vi "Main.vi"() -> ()   [LabVIEW 2014]
doc: "This sample project is built upon the standard state machine template and shows how you could create an application that acquires, analyzes, and presents data. It includes functionality for presenting configuration dialogs, preserving settings between executions, loading and saving data, as well as exporting graph images and text files.\n\nIt is most appropriate for data that is acquired instantly as it does not allow for screen updates mid acquisition nor does it allow for continuous streaming to disk."
uses:
  romtests/testproj/controls/DAQSettings.ctl
  romtests/testproj/controls/TriggerMode.ctl
  romtests/testproj/controls/AspicSettings.ctl
  romtests/testproj/controls/AspicMode.ctl
  romtests/testproj/controls/Timeslice.ctl
  romtests/testproj/controls/SystemSet.ctl
  romtests/testproj/controls/Data.ctl
  romtests/testproj/controls/UI References.ctl
  romtests/testproj/controls/Graph Data.ctl
  <vilib>/Utility/miscctls.llb/LVAnnotationListTypeDef.ctl
  <vilib>/Utility/miscctls.llb/LVCursorListTypeDef.ctl
  romtests/testproj/controls/User Specified Data.ctl
  romtests/testproj/controls/HW Configuration.ctl
  romtests/testproj/controls/Simulated Signal Type.ctl
  romtests/testproj/controls/Analysis Configuration.ctl
  romtests/testproj/controls/New Data Behavior.ctl
  romtests/testproj/controls/Network.ctl
  romtests/testproj/controls/CommSelect.ctl
  romtests/testproj/controls/State.ctl
panel:
  out "size(s)":i32[](array[numeric])
  in  "Channel":T1(ring)
  in  "Show":bool
  out "System Set":T2
  in  "SystemSet":bool
  in  "DAQSettings":bool
  in  "Timeslice":bool
  in  "Path settings":bool
  in  "Network Settings":bool
  in  "ASPIC Settings":bool
  in  "Snapshot":bool
  in  "Analyze":bool
  in  "Clear":bool
  in  "Exit":bool
  in  "Acquire":bool
  in  "Export":bool
  in  "Save Data":bool
  in  "Load Data":bool
  in  "Numeric":dbl
  out "timeslice":T3
  out "Aspic Seeting":T4 {"RC" format="%b"; "Gain" format="%b"}
  out "DAQ Settings":T6
  out "Graph":waveform(dbl)[](graph)
  out "Status Bar":string
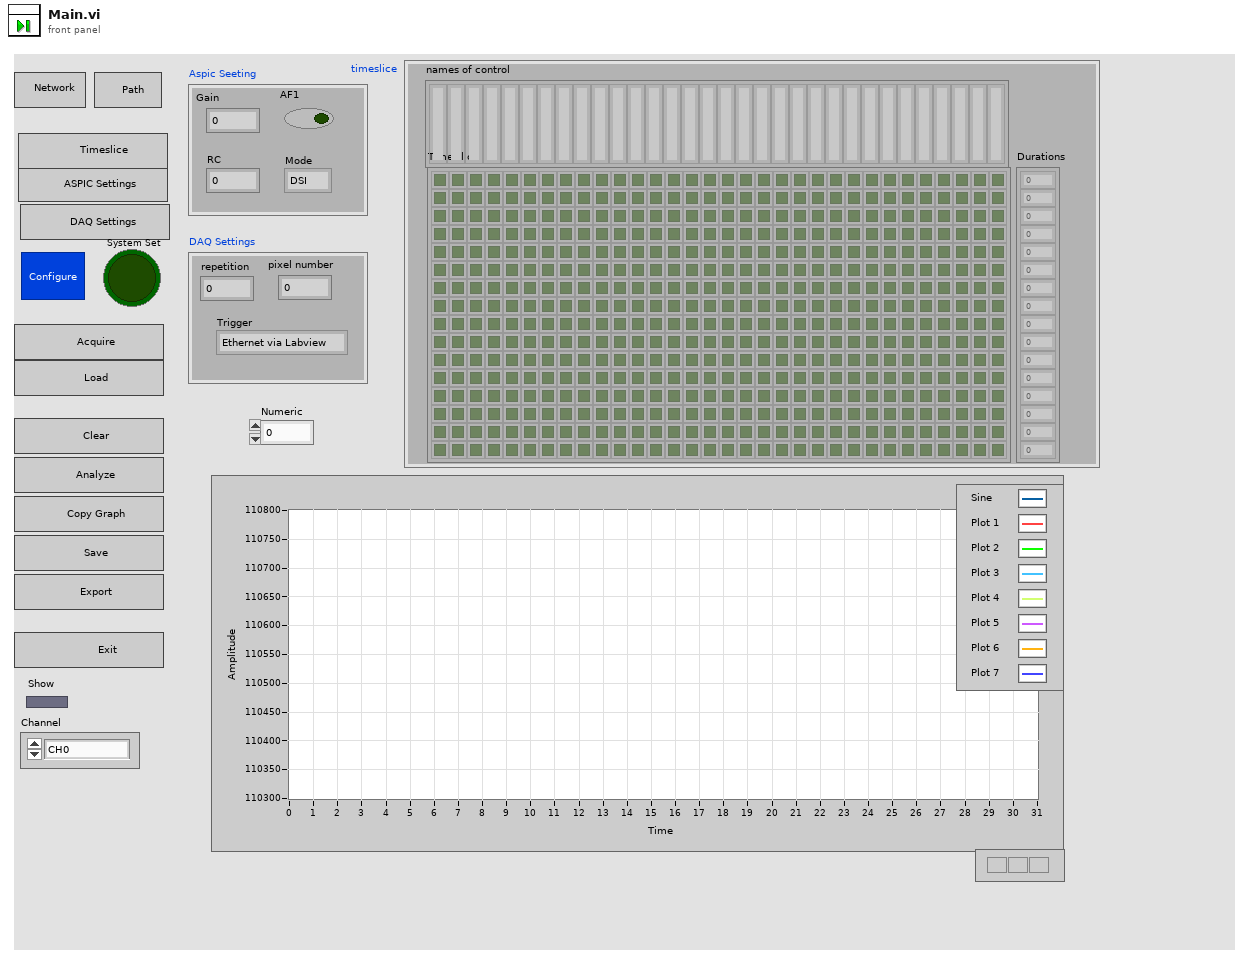
[diagram p1: front panel]
types:
  T1 = enum16{"CH0", "CH1", "CH2", "CH3", "CH4", "CH5", "CH6", "CH7", "All"}
  T2 = typedef "SystemSet.ctl" = bool
  T3 = typedef "Timeslice.ctl" = cluster{"Time slice":bool[][], "Durations":dbl[], "names of control":string[]}
  T4 = typedef "AspicSettings.ctl" = cluster{"Gain":u8, "RC":u8, "aspic1Data":u32[], "aspic2Data":u32[], "AF1":bool, "Mode":T5}
  T5 = typedef "AspicMode.ctl" = enum16{"DSI", "TM"}
  T6 = typedef "DAQSettings.ctl" = cluster{"pixel number":u32, "repetition":u32, "Trigger":T7}
  T7 = typedef "TriggerMode.ctl" = enum16{"Ethernet via Labview", "SMA (1.8V)"}
  T8 = typedef "State.ctl" = enum16{"Initialize", "Wait for Event", "Update UI", "Network", "Configure", "DAQSettings", "Timeslice", "Set Sytem", "Acquire", "Load Data", "Save Data", "Clear Data", "Export Data", "Analyze", "Copy Graph", "Exit"}
  T9 = typedef "Data.ctl" = cluster{"UI References":T10, "Graph Data":T11, "User Specified":T14, "Aspic Seeting":T4, "Network":T19, "timeslice":T3, "Acquisition Settings":T6, "CommSelect":T20, "System Set":T2}
  T10 = typedef "UI References.ctl" = cluster{"Exit Ref":refnum<vi>, "Save Ref":refnum<vi>, "Open Ref":refnum<vi>, "Export Ref":refnum<vi>, "Acquire Ref":refnum<vi>, "Configure Ref":refnum<vi>, "Graph Ref":refnum<vi>, "Clear Ref":refnum<vi>, "Analyze Ref":refnum<vi>, "Status Ref":refnum<vi>, "Snapshot Ref":refnum<vi>, "Network Ref":refnum<vi>, "Timeslice Ref":refnum<vi>, "DAQSetting Ref":refnum<vi>, "SystemSet":refnum<vi>}
  T11 = typedef "Graph Data.ctl" = cluster{"Data":waveform(dbl)[], "Annotation List":T12, "Cursor List":T13, "Analysis Data":waveform(dbl)[]}
  T12 = typedef "LVAnnotationListTypeDef.ctl" = cluster{"Name":string, "Color":u32, "Style":u8, "Point Style":u8, "Name Visible":bool, "Allow Drag":bool, "Annotation Mode":u32, "Plot":i32, "Index":i32, "Position":cluster{"X":dbl, "Y":dbl}, "X Scale":u32, "Y Scale":u32, "Show Arrow":bool, "Lock Name":bool, "Plot Area":i32, "Label Offset":cluster{"X":dbl, "Y":dbl}}[]
  T13 = typedef "LVCursorListTypeDef.ctl" = cluster{"Name":string, "Color":u32, "Style":u8, "Point Style":u8, "Name Visible":bool, "Allow Drag":bool, "Cursor Mode":u32, "Plot":i32, "Index":i32, "Position":cluster{"X":dbl, "Y":dbl}, "X Scale":u32, "Y Scale":u32, "Watch Plots":i32[], "Watch All Plots":bool, "Plot Area":i32, "Label Offset":cluster{"X":dbl, "Y":dbl}}[]
  T14 = typedef "User Specified Data.ctl" = cluster{"Hardware Configuration":T15, "Analysis Configuration":T17, "New Data Behavior":T18}
  T15 = typedef "HW Configuration.ctl" = cluster{"HW Refnum <Replace Me>":string, "Signal Type <Replace Me>":T16}
  T16 = typedef "Simulated Signal Type.ctl" = enum16{"Sine Wave", "Square Wave"}
  T17 = typedef "Analysis Configuration.ctl" = cluster{"Statistics":bool}
  T18 = typedef "New Data Behavior.ctl" = enum16{"Replace", "Overlay", "Append"}
  T19 = typedef "Network.ctl" = cluster{"invert_send":bool, "Number of datagrams to read":u32, "max bytes/read":i32, "Timeout":i32, "host":string, "Port Receive":u16}
  T20 = typedef "CommSelect.ctl" = enum16{"startTSL", "writeCABAC", "readCABAC", "resetCABAC", "emissionTest", "regRead", "executeASPIC", "resetASPIC", "resetFifo18ASPIC", "resetFifo16ASPIC", "LabviewDamicStart"}
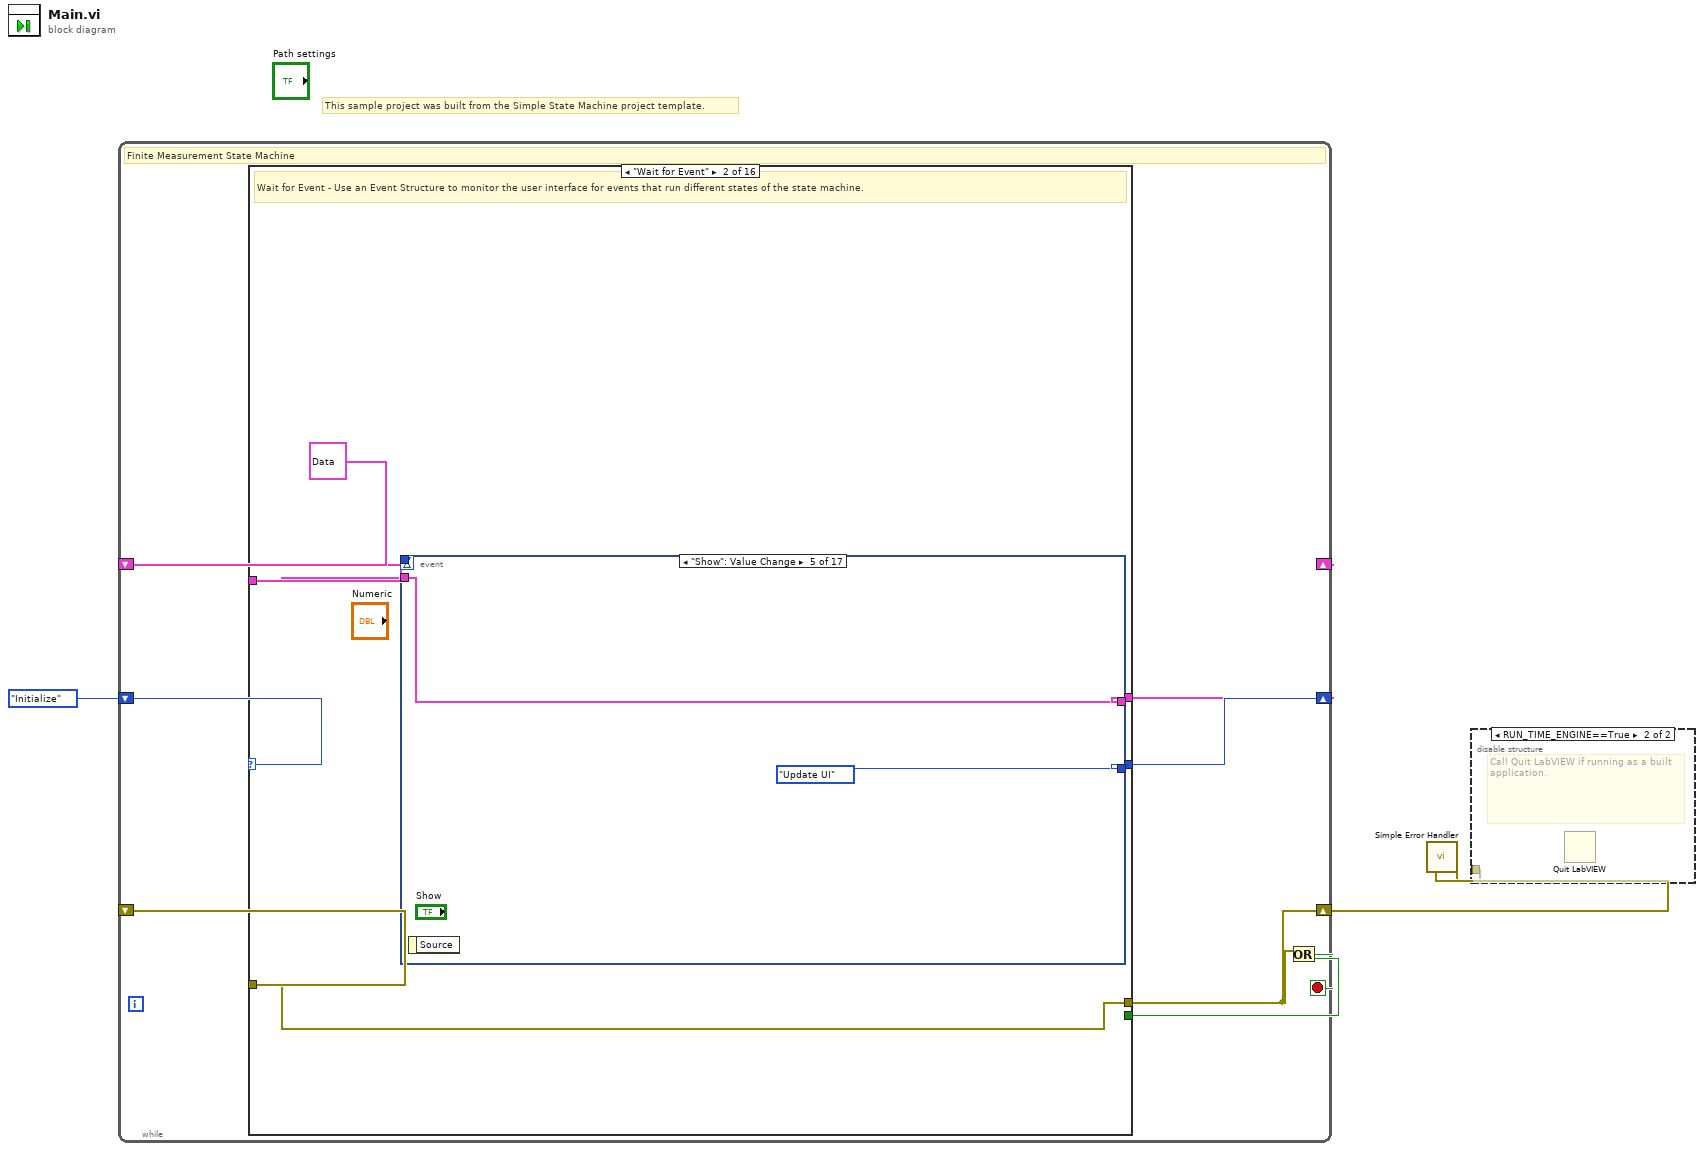
[diagram p0: block diagram]
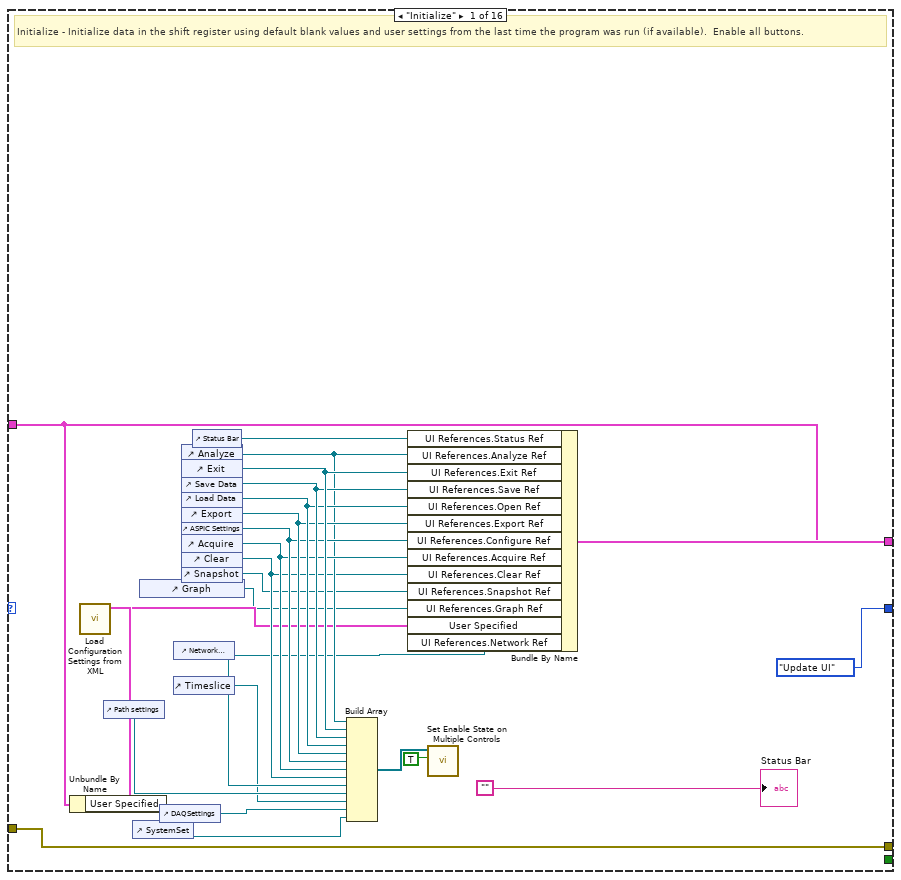
[diagram p3: hidden frame]
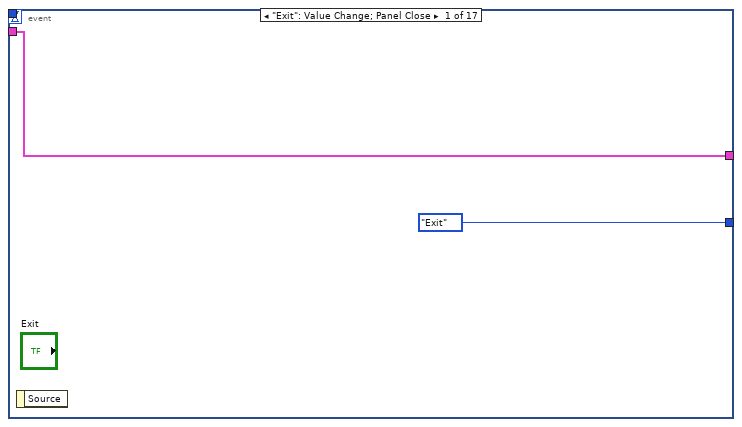
[diagram p4: hidden frame]
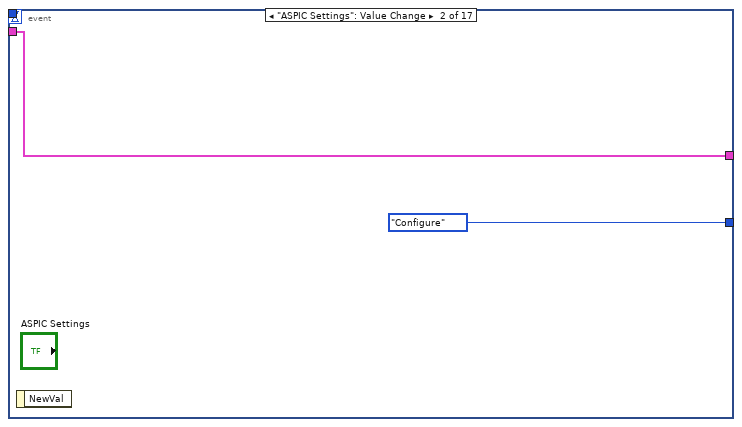
[diagram p5: hidden frame]
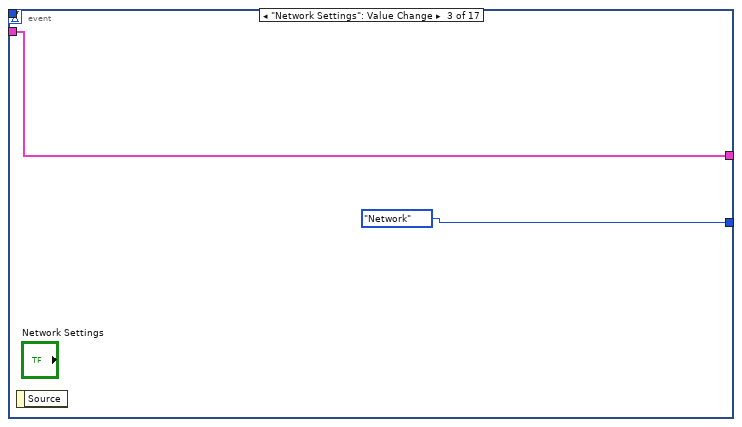
[diagram p6: hidden frame]
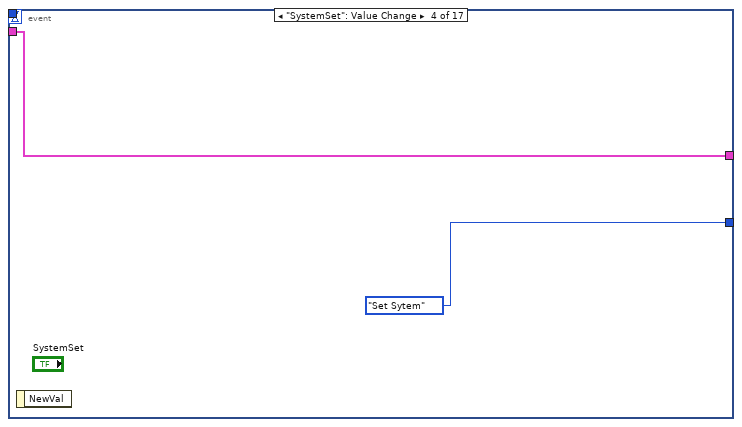
[diagram p7: hidden frame]
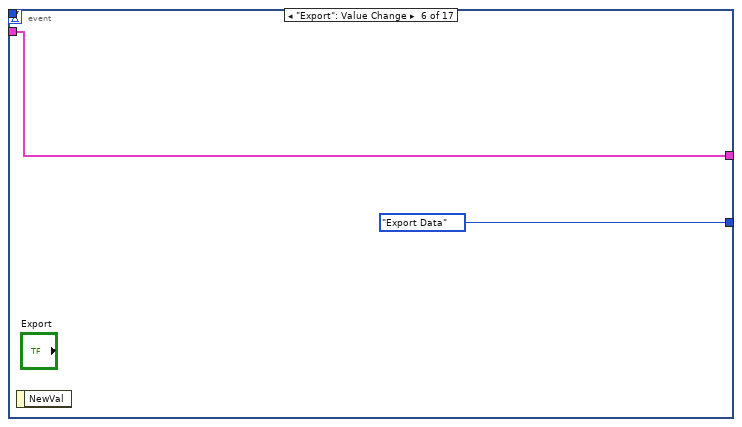
[diagram p8: hidden frame]
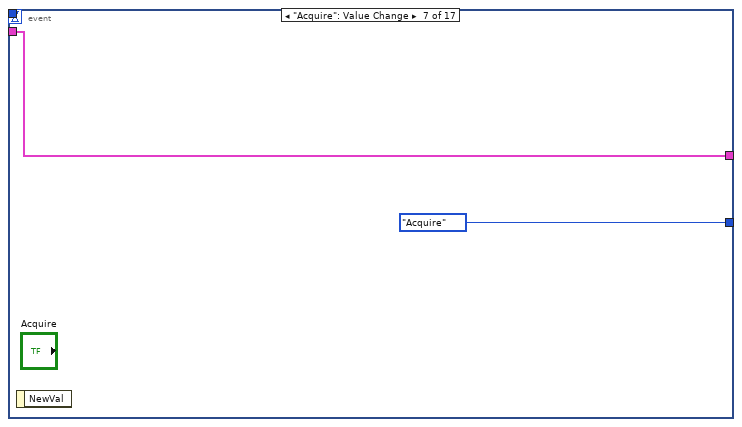
[diagram p9: hidden frame]
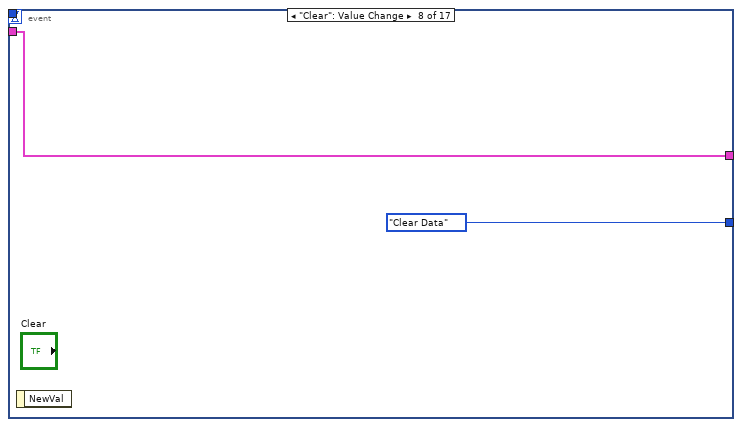
[diagram p10: hidden frame]
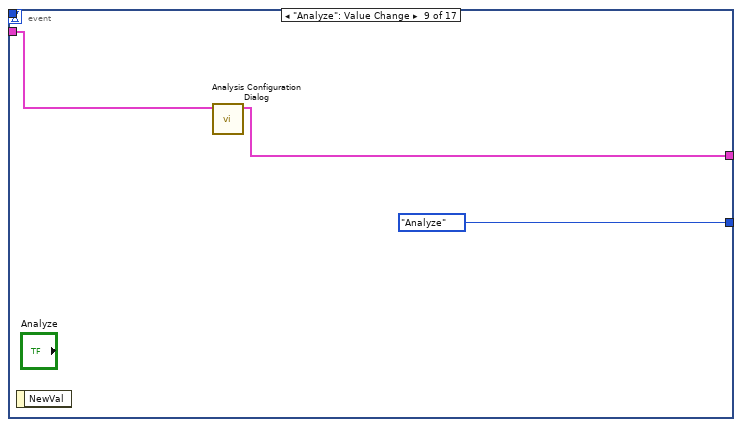
[diagram p11: hidden frame]
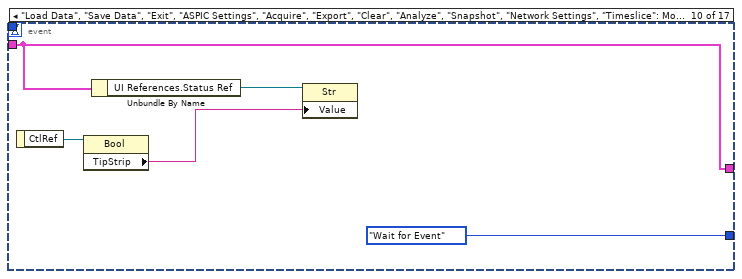
[diagram p12: hidden frame]
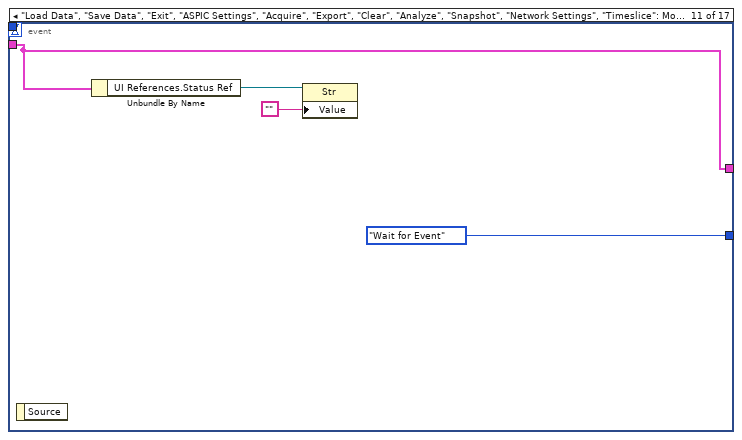
[diagram p13: hidden frame]
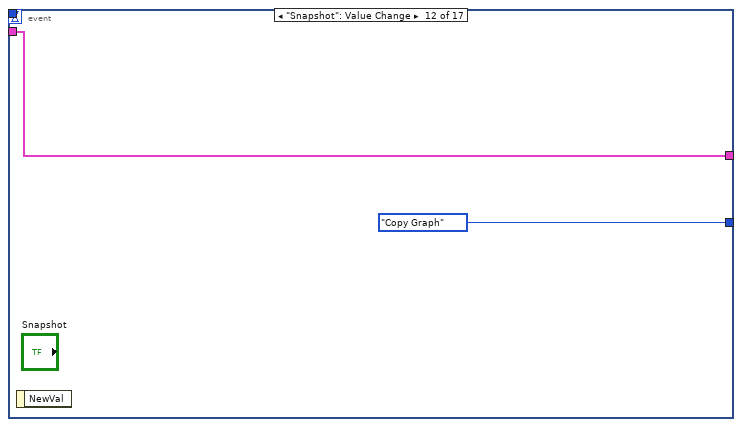
[diagram p14: hidden frame]
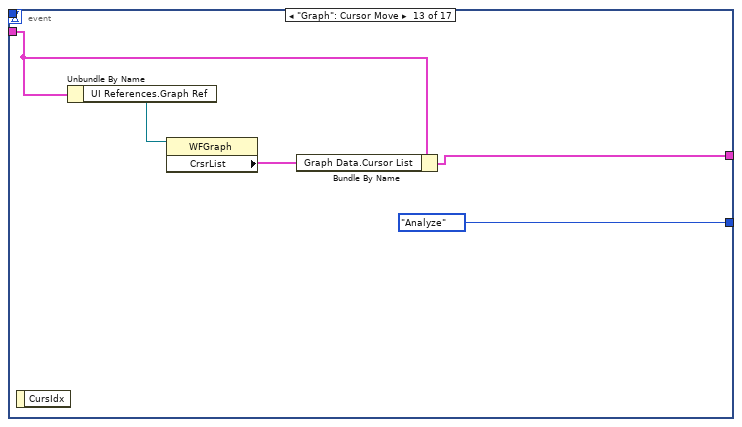
[diagram p15: hidden frame]
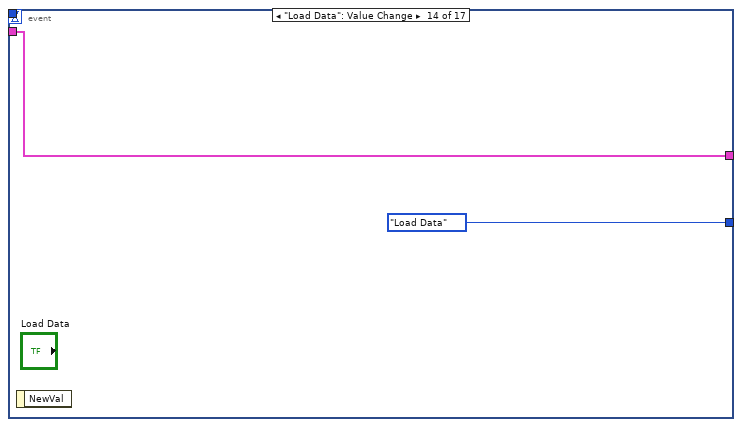
[diagram p16: hidden frame]
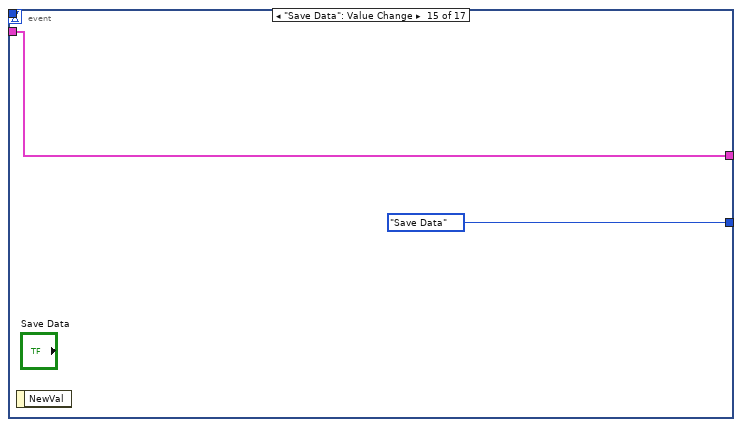
[diagram p17: hidden frame]
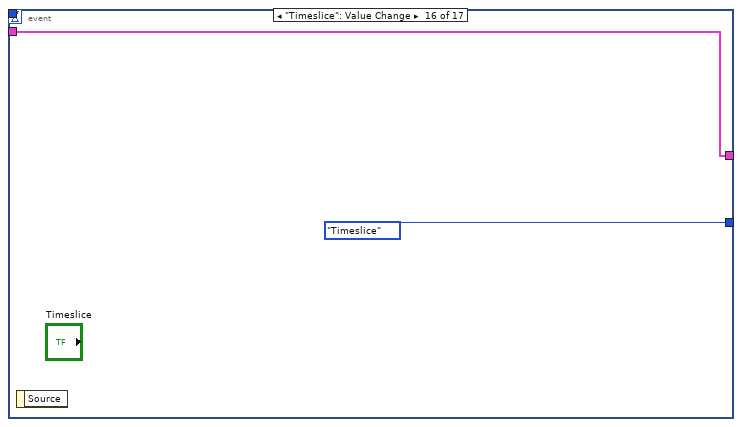
[diagram p18: hidden frame]
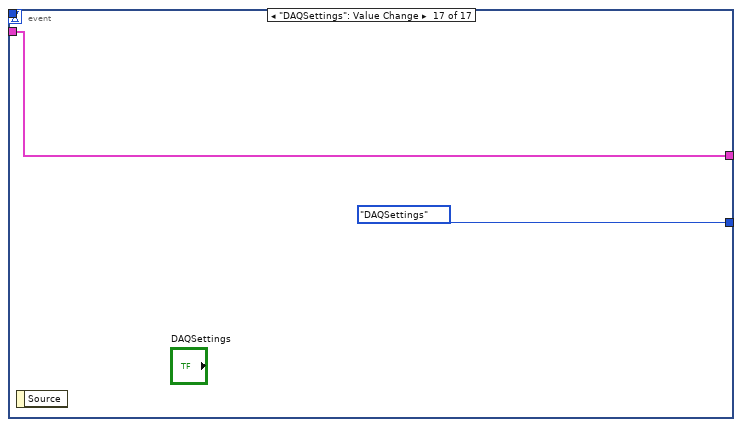
[diagram p19: hidden frame]
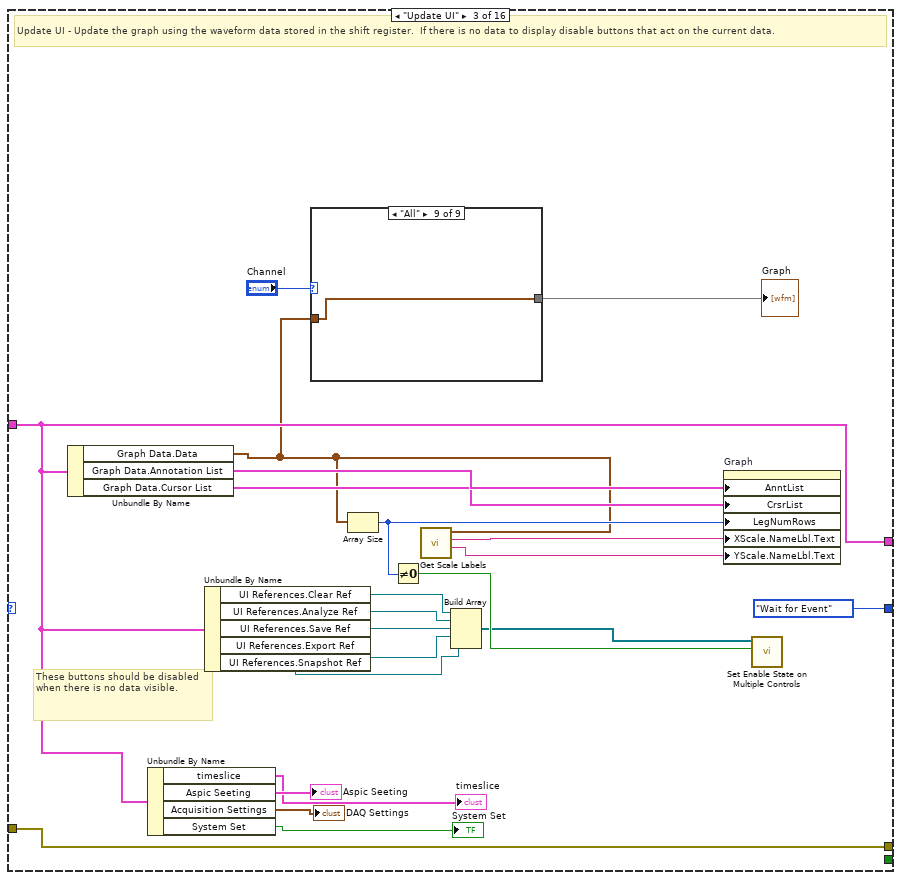
[diagram p20: hidden frame]
diagram:
  # "This sample project was built from the Simple State Machine project template."
  n1 = while {
    shift-right: [w11] -> _
    shift-left: State."Initialize" ("Next State") -> [w12]
    shift-right: [w5] -> w4
    shift-left: _ -> [w6]
    shift-right: [w7] -> _
    shift-left: T9 {"UI References"={"Exit Ref"=refnum, "Save Ref"=refnum, "Open Ref"=refnum, "Export Ref"=refnum, "Acquire Ref"=refnum, "Configure Ref"=refnum, "Graph Ref"=refnum, "Clear Ref"=refnum, "Analyze Ref"=refnum, "Status Ref"=refnum, "Snapshot Ref"=refnum, "Network Ref"=refnum, "Timeslice Ref"=refnum, "DAQSetting Ref"=refnum, "SystemSet"=refnum}, "Graph Data"={"Data"=[], "Annotation List"=[], "Cursor List"=[], "Analysis Data"=[]}, "User Specified"={"Hardware Configuration"={"HW Refnum <Replace Me>"="", "Signal Type <Replace Me>"=enum."Sine Wave"}, "Analysis Configuration"={"Statistics"=TRUE}, "New Data Behavior"=enum."Replace"}, "Aspic Seeting"={"Gain"=0, "RC"=0, "aspic1Data"=[], "aspic2Data"=[], "AF1"=FALSE, "Mode"=enum."TM"}, "Network"={"invert_send"=TRUE, "Number of datagrams to read"=5000, "max bytes/read"=2500, "Timeout"=4000, "host"="192.168.1.18", "Port Receive"=5678}, "timeslice"={"Time slice"=[], "Durations"=[], "names of control"=[]}, "Acquisition Settings"={"pixel number"=0, "repetition"=0, "Trigger"=enum."Ethernet via Labview"}, "CommSelect"=enum."resetFifo18ASPIC", "System Set"=FALSE} ("Data") -> [w8]
    stop <- w9 stop-if-true
    # "Finite Measurement State Machine"
    n2 = case shown="\"Wait for Event\"" w12 {
      tunnel: [State."Update UI" ("Next State") w41 State."Wait for Event" ("(Value Not Used)") w125 State."Update UI" ("Next State if true") State."Update UI" ("Next State if true") w161 State."Update UI" ("States") State."Update UI" ("Next State") State."Update UI" ("(Value Not Used)") State."Wait for Event" ("(Value Not Used)") State."Wait for Event" ("(Value Not Used)") State."Update UI" ("(Value Not Used)") State."Update UI" ("(Value Not Used)") State."Wait for Event" ("(Value Not Used)") w284] -> w11
      tunnel: [_ _ _ _ _ _ _ _ _ _ _ _ _ _ _ w283] -> w10
      tunnel: w8 -> [w17 w40 w93 w131 w143 w150 w159 w175 w202 w223 w240 w253 w266 w270 w275 w279]
      tunnel: [w18 w39 w93 w130 w135 w144 w153 w171 w195 w222 w240 w253 w265 w270 w275 w279] -> w7
      tunnel: w6 -> [w16 w38 w94 w127 w142 w149 w165 w173 w201 w220 w239 w252 w264 w269 w274 w278]
      tunnel: [w16 w38 w94 w126 w139 w148 w165 w166 w200 w219 w238 w251 w264 w269 w273 w277] -> w5
      frame "Initialize" {
        # "Initialize - Initialize data in the shift register using default blank values and user settings from the last time the program was run (if available).  Enable all buttons."
        n3 = Unbundle By Name(w17) -> ("User Specified"=w29:T14)
        n4 = call "Load Configuration Settings from XML.vi"("User Configuration in"=w29) -> ("User Configuration out"=w24:T14)  [unwired: 9 in, 1 out]
        n5 = control-ref of="Path settings"() -> (w20:refnum<vi>)
        n6 = control-ref of="SystemSet"() -> (w13:refnum<vi>)
        n7 = control-ref of="Graph"() -> (w21:refnum<vi>)
        n8 = control-ref of="DAQSettings"() -> (w14:refnum<vi>)
        n9 = control-ref of="Network Settings"() -> (w19:refnum<vi>)
        n10 = control-ref of="Timeslice"() -> (w15:refnum<vi>)
        n11 = control-ref of="Analyze"() -> (w28:refnum<vi>)
        n12 = control-ref of="Exit"() -> (w36:refnum<vi>)
        n13 = control-ref of="Save Data"() -> (w35:refnum<vi>)
        n14 = control-ref of="Load Data"() -> (w34:refnum<vi>)
        n15 = control-ref of="Export"() -> (w33:refnum<vi>)
        n16 = control-ref of="ASPIC Settings"() -> (w32:refnum<vi>)
        n17 = control-ref of="Acquire"() -> (w31:refnum<vi>)
        n18 = control-ref of="Clear"() -> (w26:refnum<vi>)
        n19 = control-ref of="Snapshot"() -> (w22:refnum<vi>)
        n20 = control-ref of="Status Bar"() -> (w27:refnum<vi>)
        n21 = Build Array(w28, w36, w35, w34, w33, w32, w31, w26, w19, w20, w15, w14, w13) -> (w30:refnum<vi>[])
        n22 = Bundle By Name(cluster=w17, "UI References.Status Ref"=w27, "UI References.Analyze Ref"=w28, "UI References.Exit Ref"=w36, "UI References.Save Ref"=w35, "UI References.Open Ref"=w34, "UI References.Export Ref"=w33, "UI References.Configure Ref"=w32, "UI References.Acquire Ref"=w31, "UI References.Clear Ref"=w26, "UI References.Snapshot Ref"=w22, "UI References.Graph Ref"=w21, "User Specified"=w24, "UI References.Network Ref"=w19) -> (w18:T9)
        n23 = call "Set Enable State on Multiple Controls.vi"("Enable?"=TRUE, "Controls"=w30) -> ()  [unwired: 10 in]
        "Status Bar" <- "" ("Status Bar")
      }
      frame "Wait for Event" {
        # "Wait for Event - Use an Event Structure to monitor the user interface for events that run different states of the state machine."
        n24 = event shown="[4] \"Show\": Value Change" {
          selector: _ -> [_ _ _ _ _ _ _ _ _ _ _ _ _ _ _ _ _]
          dyn-events: _ -> [_ _ _ _ _ _ _ _ _ _ _ _ _ _ _ _ _]
          timeout: _ -> [_ w45 _ _ _ _ _ _ _ _ _ _ _ _ _ _ _]
          tunnel: [State."Exit" ("Next State") State."Configure" ("Next State") State."Network" ("States") State."Set Sytem" ("States") State."Update UI" ("States") State."Export Data" ("Next State") State."Acquire" ("Next State") State."Clear Data" ("Next State") State."Analyze" ("Next State") State."Wait for Event" ("Next State") State."Wait for Event" ("Next State") State."Copy Graph" ("Next State") State."Analyze" ("Next State") State."Load Data" ("Next State") State."Save Data" ("Next State") State."Timeslice" ("States") State."DAQSettings" ("States")] -> w41
          tunnel: [_ w45 _ _ _ _ _ _ _ _ _ _ _ _ _ _ _] -> _
          tunnel: w40 -> [w42 w44 w48 w50 w52 w53 w55 w57 w60 w62 w67 w71 w74 w78 w80 w83 w85]
          tunnel: [w42 w44 w48 w50 w52 w53 w55 w57 w59 w62 w67 w71 w73 w78 w80 w83 w85] -> w39
          event "Exit": Value Change; Panel Close {
            n25 = event-data() -> ()  [unwired: 1 in, 1 out]
          }
          event "ASPIC Settings": Value Change {
            n26 = event-data() -> ()  [unwired: 1 in, 1 out]
          }
          event "Network Settings": Value Change {
            n27 = event-data() -> ()  [unwired: 1 in, 1 out]
          }
          event "SystemSet": Value Change {
            n28 = event-data() -> ()  [unwired: 1 in, 1 out]
          }
          event "Show": Value Change {
            n29 = event-data() -> ()  [unwired: 1 in, 1 out]
          }
          event "Export": Value Change {
            n30 = event-data() -> ()  [unwired: 1 in, 1 out]
          }
          event "Acquire": Value Change {
            n31 = event-data() -> ()  [unwired: 1 in, 1 out]
          }
          event "Clear": Value Change {
            n32 = event-data() -> ()  [unwired: 1 in, 1 out]
          }
          event "Analyze": Value Change {
            n33 = event-data() -> ()  [unwired: 1 in, 1 out]
            n34 = call "Analysis Configuration Dialog.vi"("Data In"=w60) -> ("Data out"=w59:T9)  [unwired: 10 in]
          }
          event "Load Data", "Save Data", "Exit", "ASPIC Settings", "Acquire", "Export", "Clear", "Analyze", "Snapshot", "Network Settings", "Timeslice": Mouse Enter {
            n35 = event-data() -> ("CtlRef"=w66:refnum<vi>)  [unwired: 1 in]
            n36 = property class="Bool"(reference=w66) -> ("TipStrip"=w64:string)  [unwired: 1 in, 2 out]
            n37 = Unbundle By Name(w62) -> ("UI References.Status Ref"=w65:refnum<vi>)
            n38 = property class="Str"(reference=w65, "Value"=w64) -> ()  [unwired: 1 in, 2 out]
          }
          event "Load Data", "Save Data", "Exit", "ASPIC Settings", "Acquire", "Export", "Clear", "Analyze", "Snapshot", "Network Settings", "Timeslice": Mouse Leave {
            n39 = event-data() -> ()  [unwired: 1 in, 1 out]
            n40 = Unbundle By Name(w67) -> ("UI References.Status Ref"=w70:refnum<vi>)
            n41 = property class="Str"(reference=w70, "Value"="") -> ()  [unwired: 1 in, 2 out]
          }
          event "Snapshot": Value Change {
            n42 = event-data() -> ()  [unwired: 1 in, 1 out]
          }
          event "Graph": Cursor Move {
            n43 = event-data() -> ()  [unwired: 1 in, 1 out]
            n44 = Unbundle By Name(w74) -> ("UI References.Graph Ref"=w76:refnum<vi>)
            n45 = property class="WFGraph"(reference=w76) -> ("CrsrList"=w75:T13)  [unwired: 1 in, 2 out]
            n46 = Bundle By Name(cluster=w74, "Graph Data.Cursor List"=w75) -> (w73:T9)
          }
          event "Load Data": Value Change {
            n47 = event-data() -> ()  [unwired: 1 in, 1 out]
          }
          event "Save Data": Value Change {
            n48 = event-data() -> ()  [unwired: 1 in, 1 out]
          }
          event "Timeslice": Value Change {
            n49 = event-data() -> ()  [unwired: 1 in, 1 out]
          }
          event "DAQSettings": Value Change {
            n50 = event-data() -> ()  [unwired: 1 in, 1 out]
          }
        }
      }
      frame "Update UI" {
        # "These buttons should be disabled when there is no data visible."
        # "Update UI - Update the graph using the waveform data stored in the shift register.  If there is no data to display disable buttons that act on the current data."
        n51 = Unbundle By Name(w93) -> ("Graph Data.Data"=w87:waveform(dbl)[], "Graph Data.Annotation List"=w97:T12, "Graph Data.Cursor List"=w96:T13)
        n52 = Unbundle By Name(w93) -> ("timeslice"=→"timeslice":T3, "Aspic Seeting"=→"Aspic Seeting":T4, "Acquisition Settings"=→"DAQ Settings":T6, "System Set"=→"System Set":T2)
        n53 = Unbundle By Name(w93) -> ("UI References.Clear Ref"=w103:refnum<vi>, "UI References.Analyze Ref"=w102:refnum<vi>, "UI References.Save Ref"=w106:refnum<vi>, "UI References.Export Ref"=w100:refnum<vi>, "UI References.Snapshot Ref"=w101:refnum<vi>)
        n54 = case shown="\"All\"" "Channel" {
          tunnel: w87 -> [w109 w111 w113 w115 w117 w119 w121 w123 w124]
          tunnel: [w108 w110 w112 w114 w116 w118 w120 w122 w124] -> w86
          frame "CH0", Default {
            n55 = Decimate 1D Array(w109) -> (w108:waveform(dbl)[])  [unwired: 7 out]
          }
          frame "CH1" {
            n56 = Decimate 1D Array(w111) -> (w110:waveform(dbl)[])  [unwired: 7 out]
          }
          frame "CH2" {
            n57 = Decimate 1D Array(w113) -> (w112:waveform(dbl)[])  [unwired: 7 out]
          }
          frame "CH3" {
            n58 = Decimate 1D Array(w115) -> (w114:waveform(dbl)[])  [unwired: 7 out]
          }
          frame "CH4" {
            n59 = Decimate 1D Array(w117) -> (w116:waveform(dbl)[])  [unwired: 7 out]
          }
          frame "CH5" {
            n60 = Decimate 1D Array(w119) -> (w118:waveform(dbl)[])  [unwired: 7 out]
          }
          frame "CH6" {
            n61 = Decimate 1D Array(w121) -> (w120:waveform(dbl)[])  [unwired: 7 out]
          }
          frame "CH7" {
            n62 = Decimate 1D Array(w123) -> (w122:waveform(dbl)[])  [unwired: 7 out]
          }
          frame "All" {
          }
        }
        "Graph" <- w86
        n63 = Array Size(array=w87) -> (size(s)=w105:i32)
        n64 = Not Equal To 0?(x=w105) -> (x != 0?=w104:bool)
        n65 = call "Get Scale Labels.vi"("Array of Waveforms"=w87) -> ("Y Scale Label Text"=w98:string, "X Scale Label Text"=w99:string)  [unwired: 9 in]
        n66 = Build Array(w103, w102, w106, w100, w101) -> (w95:refnum<vi>[])
        n67 = property on="Graph" class="WFGraph (strict)"("AnntList"=w97, "CrsrList"=w96, "LegNumRows"=w105, "XScale.NameLbl.Text"=w99, "YScale.NameLbl.Text"=w98) -> ()  [unwired: 2 in, 2 out]
        n68 = call "Set Enable State on Multiple Controls.vi"("Enable?"=w104, "Controls"=w95) -> ()  [unwired: 10 in]
      }
      frame "Network" {
        n69 = Unbundle By Name(w131) -> ("Network"=w132:T19)
        n70 = call "NetworkSettingsDialog.vi"("error in (no error)"=w127, "Network In"=w132) -> ("error out"=w126:errorcluster, "UI Refresh Needed?"=w128:bool, "Network Out"=w129:T19)  [unwired: 7 in]
        n71 = Bundle By Name(cluster=w131, "Network"=w129) -> (w130:T9)
        n72 = Select(t=State."Update UI" ("Next State if true"), s=w128, f=State."Wait for Event" ("Next State if false")) -> (s? t:f=w125:T8)
      }
      frame "Configure" {
        # "Configure - Spawns a dialog that allows the user to set any user configurable settings."
        n73 = Unbundle By Name(w143) -> ("Aspic Seeting"=w141:T4)
        n74 = call "AspicSettingsDialog.vi"("error in (no error)"=w142, "Aspic Seeting In"=w141) -> ("error out"=w139:errorcluster, "Aspic Seeting Out"=w140:T4)  [unwired: 5 in, 1 out]
        n75 = Bundle By Name(cluster=w143, "Aspic Seeting"=w140) -> (w136:T9)
        n76 = Bundle By Name(cluster=w136, "System Set"=FALSE) -> (w135:T9)
      }
      frame "DAQSettings" {
        n77 = Unbundle By Name(w150) -> ("Acquisition Settings"=w152:T6)
        n78 = call "DAQSettingsDialog.vi"("error in (no error)"=w149, "Acquisition Settings In"=w152) -> ("error out"=w148:errorcluster, "Acquisition Settings Out"=w151:T6)  [unwired: 7 in, 1 out]
        n79 = Bundle By Name(cluster=w150, "Acquisition Settings"=w151) -> (w145:T9)
        n80 = Bundle By Name(cluster=w145, "System Set"=FALSE) -> (w144:T9)
      }
      frame "Timeslice" {
        n81 = Unbundle By Name(w159) -> ("timeslice"=w160:T3)
        n82 = call "SetTimesliceDialog.vi"("timeslice in"=w160) -> ("timeslice out"=w158:T3)  [unwired: 10 in]
        n83 = Bundle By Name(cluster=w159, "timeslice"=w158) -> (w154:T9)
        n84 = Unbundle By Name(w154) -> ("timeslice.Time slice"=w157:bool[][])
        n85 = Array Size(array=w157) -> (size(s)=→"size(s)":i32[])
        n86 = Select(t=State."Update UI" ("Next State if true"), s=TRUE, f=State."Wait for Event" ("Next State if false")) -> (s? t:f=w161:T8)
        n87 = Bundle By Name(cluster=w154, "System Set"=FALSE) -> (w153:T9)
      }
      frame "Set Sytem" {
        # "reset the FIFO of the FPGA"
        # "ASPIC gain / RC etc"
        n88 = flat-sequence {
          tunnel: w175 -> [w180]
          tunnel: [w178] -> w174
          tunnel: w173 -> [_]
          tunnel: [w177] -> w172
          tunnel: w174 -> [w187]
          tunnel: w172 -> [w186]
          tunnel: [w187] -> w169
          tunnel: [w182] -> w167
          tunnel: w169 -> [w189]
          tunnel: [w189] -> w168
          tunnel: w167 -> [w188]
          tunnel: [w188] -> w166
          tunnel: [w192] -> w171
          tunnel: w168 -> [w194]
          frame #0 {
            n89 = Unbundle By Name(w180) -> ("Aspic Seeting"=w181:T4, "Acquisition Settings"=w176:T6)
            n90 = call "SetASPIC.vi"("Acquisition Settings"=w176, "Aspic Seeting In"=w181) -> ("error out"=w177:errorcluster, "Aspic Seeting Out"=w179:T4)  [unwired: 8 in]
            n91 = Bundle By Name(cluster=w180, "Aspic Seeting"=w179) -> (w178:T9)
          }
          frame #1 {
            n92 = call "programComm.vi"("error in (no error)"=w186, "CommSelect"=CommSelect."resetFifo16ASPIC") -> ("error out"=w183:errorcluster)
            n93 = call "programComm.vi"("error in (no error)"=w183, "CommSelect"=CommSelect."resetFifo18ASPIC") -> ("error out"=w182:errorcluster)
          }
          frame #2 {
            n94 = Unbundle By Name(w189) -> ("timeslice"=w191:T3, "Acquisition Settings"=w190:T6)
            n95 = call "SetTS.vi"("Acquisition Settings"=w190, "timeslice"=w191) -> ()  [unwired: 10 in]
          }
          frame #3 {
            n96 = Bundle By Name(cluster=w194, "System Set"=TRUE) -> (w192:T9)
          }
        }
      }
      frame "Acquire" {
        # "Acquire - Uses the current hardware configuration to acquire a new data set and stores it in the state data."
        n97 = Unbundle By Name(w202) -> ("UI References.Status Ref"=w203:refnum<vi>, "Acquisition Settings"=w207:T6, "Network"=w199:T19)
        n98 = call "Acquire Data from Hardware.vi"("error in (no error)"=w201, "read"=TRUE, "Network"=w199, "Acquisition Settings"=w207) -> ("error out"=w204:errorcluster, "Graph Data 2"=w196:T11, "Graph Data"=w205:waveform(dbl)[])  [unwired: 5 in]
        n99 = case shown="No Error" w204 {
          selector: w204 -> [w212 w218]
          tunnel: [w214 w216] -> w197
          tunnel: w205 -> [w213 _]
          tunnel: ["Data acquired." ("Data acquired") "Data not acquired." ("Data not acquired")] -> w206
          tunnel: w202 -> [w210 w216]
          tunnel: [w209 w215] -> w200
          frame No Error {
            n100 = call "Incorporate New Data.vi"("error in (no error)"=w212, "New Graph Data"=w213, "Data in"=w210) -> ("error out"=w209:errorcluster, "Data out"=w214:T9)  [unwired: 7 in]
          }
          frame Error {
            n101 = call <vilib>:"Simple Error Handler.vi"("error in (no error)"=w218) -> ("error out"=w215:errorcluster)  [unwired: 4 in, 4 out]
          }
        }
        n102 = property class="Str"(reference=w203, "Value"=w206) -> ()  [unwired: 1 in, 2 out]
        n103 = Bundle By Name(cluster=w197, "Graph Data"=w196) -> (w195:T9)
      }
      frame "Load Data" {
        # "Load Data - Loads data from a TDMS file and incorporates it with the existing data according to the user's preference."
        n104 = call "Load Data.vi"("error in (no error)"=w220) -> ("error out"=w226:errorcluster, "New Graph Data"=w224:waveform(dbl)[])  [unwired: 9 in]
        n105 = case shown="No Error" w226 {
          selector: w226 -> [w231 w237]
          tunnel: [w233 w235] -> w222
          tunnel: w224 -> [w232 _]
          tunnel: ["Data loaded." ("Data loaded") "Data not loaded." ("Data not loaded")] -> w225
          tunnel: w223 -> [w229 w235]
          tunnel: [w228 w234] -> w219
          frame No Error {
            n106 = call "Incorporate New Data.vi"("error in (no error)"=w231, "New Graph Data"=w232, "Data in"=w229) -> ("error out"=w228:errorcluster, "Data out"=w233:T9)  [unwired: 7 in]
          }
          frame Error {
            n107 = call <vilib>:"Simple Error Handler.vi"("error in (no error)"=w237) -> ("error out"=w234:errorcluster)  [unwired: 4 in, 4 out]
          }
        }
        n108 = Unbundle By Name(w222) -> ("UI References.Status Ref"=w221:refnum<vi>)
        n109 = property class="Str"(reference=w221, "Value"=w225) -> ()  [unwired: 1 in, 2 out]
      }
      frame "Save Data" {
        # "Save Data - Saves the existing measurement data to a TDMS file."
        n110 = Unbundle By Name(w240) -> ("UI References.Status Ref"=w241:refnum<vi>, "Graph Data.Data"=w242:waveform(dbl)[])
        n111 = call "Save Data.vi"("error in (no error)"=w239, "Data"=w242) -> ("error out"=w244:errorcluster)  [unwired: 9 in]
        n112 = case shown="Error" w244 {
          selector: w244 -> [w246 w250]
          tunnel: ["Data saved." ("Data saved") "Data not saved." ("Data not saved")] -> w243
          tunnel: [w246 w248] -> w238
          frame No Error {
          }
          frame Error {
            n113 = call <vilib>:"Simple Error Handler.vi"("error in (no error)"=w250) -> ("error out"=w248:errorcluster)  [unwired: 4 in, 4 out]
          }
        }
        n114 = property class="Str"(reference=w241, "Value"=w243) -> ()  [unwired: 1 in, 2 out]
      }
      frame "Export Data" {
        # "Export Data - Exports the currently loaded measurement and analysis data to a text file that can be imported into a spreadsheet or other application."
        n115 = Unbundle By Name(w253) -> ("UI References.Status Ref"=w254:refnum<vi>, "Graph Data"=w255:T11)
        n116 = call "Export Data.vi"("error in (no error)"=w252, "Graph Data"=w255) -> ("error out"=w256:errorcluster)  [unwired: 9 in]
        n117 = case shown="No Error" w256 {
          selector: w256 -> [w259 w263]
          tunnel: ["Data exported." ("Data exported") "Data not exported." ("Data not exported")] -> w257
          tunnel: [w259 w261] -> w251
          frame No Error {
          }
          frame Error {
            n118 = call <vilib>:"Simple Error Handler.vi"("error in (no error)"=w263) -> ("error out"=w261:errorcluster)  [unwired: 4 in, 4 out]
          }
        }
        n119 = property class="Str"(reference=w254, "Value"=w257) -> ()  [unwired: 1 in, 2 out]
      }
      frame "Clear Data" {
        # "Clear Data - Clears the data currently in the graph."
        n120 = Bundle By Name(cluster=w266, "Graph Data"=T11 {"Data"=[], "Annotation List"=[], "Cursor List"=[], "Analysis Data"=[]} ("Graph")) -> (w265:T9)
      }
      frame "Analyze" {
        # "#CodeRecommended - Add your own signal analysis here."
        # "Analyze - Analyzes the measurement data."
        n121 = Unbundle By Name(w270) -> ("Graph Data"=w271:T11)
        n122 = call "Statistical Analysis.vi"("Graph Data In"=w271) -> ()  [unwired: 9 in, 2 out]
      }
      frame "Copy Graph" {
        # "Copy Graph - Places an image of the graph on the clipboard for pasting into reports or emails."
        n123 = call "Copy Graph to Clipboard.vi"("error in (no error)"=w274, "Graph Data"=w275) -> ("error out"=w273:errorcluster)  [unwired: 9 in]
      }
      frame "Exit" {
        w283 = TRUE  # Stop Loop?
        w284 = State."Exit"  # (Value Not Used)
        # "Exit - Saves the user's settings to an XML file and stops execution."
        n124 = Unbundle By Name(w279) -> ("UI References.Status Ref"=w280:refnum<vi>, "User Specified"=w281:T14)
        n125 = call "Save Configuration Settings to XML.vi"("error in (no error)"=w278, "User Configuration"=w281) -> ("error out"=w277:errorcluster)  [unwired: 9 in]
        n126 = property class="Str"(reference=w280, "Value"="Application exit." ("Stopped")) -> ()  [unwired: 1 in, 2 out]
      }
    }
    n127 = Or(x=w5, y=w10) -> (x .or. y?=w9:bool)
  }
  n128 = call <vilib>:"Simple Error Handler.vi"("error in (no error)"=w4) -> ("error out"=w3:errorcluster)  [unwired: 4 in, 4 out]
  n129 = disable-structure shown="RUN_TIME_ENGINE==True" {
    disable-tunnel: w3 -> [_ _]
    frame condition #0 (active) {
    }
    frame condition #1 {
      # "Call Quit LabVIEW if running as a built application."
      n130 = Quit LabVIEW() -> ()  [unwired: 1 in]
    }
  }
